vi "超标留样自动校时.vi"   [LabVIEW 2016, in "德润DR803L超标留样.lvlib"]
types:
  T1 = enum16{"open", "read", "write", "write single", "close"}
  T2 = cluster{"采样器状态":enum16{"停止", "运行"}, "当前留样瓶编号":u16, "报警状态":enum16{"无报警", "缺水报警"}, "超标信号":enum16{"无信号", "超标信号"}, "采样器进程":enum16{"停止", "待机", "定位校正", "移除瓶盖", "采样瓶排空", "管路润洗", "管存", "进样", "瓶盖密封", "管路排空", "调整采样位置", "采样结束", "采样瓶润洗", "瓶润洗排空"}, "版本号":string, "同步信号":enum16{"无信号", "同步信号"}, "外控信号":enum16{"无信号", "外控信号"}, "门状态":enum16{"门开", "门关"}, "当前瓶号":u16, "工作状态":enum16{"停止", "采样中"}, "留样模式":enum16{"无", "定时留样", "时间等比例", "超标留样", "同步留样", "外控留样"}, "立即留样":enum16{"无", "远程留样"}, "采样方式":enum16{"单采", "双重"}, "仪器时间":timestamp, "单次采样量":u16, "时间等比采样采样间隔":u16, "排空命令":u16, "远程复位":u16, "门禁密码":u16}
  T3 = typedef "LVDateTimeRec.ctl" = cluster{"秒数的小数部分":dbl, "秒":i32, "分":i32, "时":i32, "日":i32, "月":i32, "年":i32, "天数（周）":i32, "天数（年）":i32, "DST":i32}
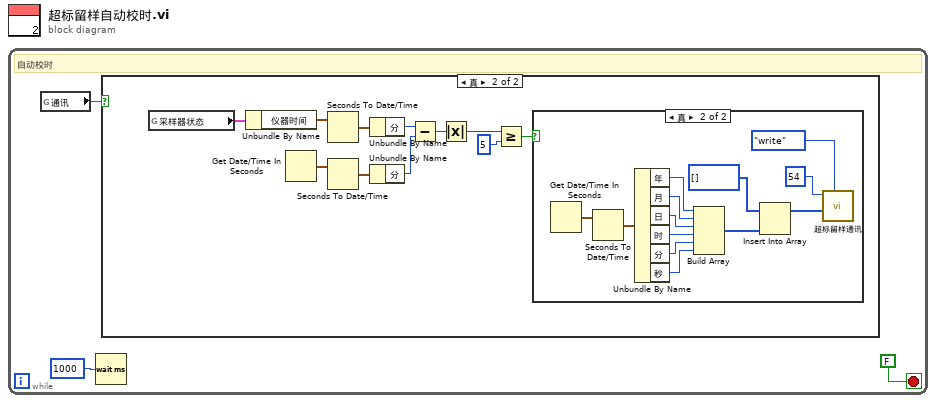
[diagram p0: block diagram]
diagram:
  n1 = while {
    stop <- FALSE stop-if-true
    # "自动校时"
    n2 = global read "超标留样全局.vi" "通讯"() -> (w1:bool)
    n3 = Wait (ms)(milliseconds to wait=u32 1000 ("等待时间（毫秒）")) -> ()  [unwired: 1 out]
    n4 = case shown="真" w1 {
      frame False {
      }
      frame True {
        n5 = global read "超标留样全局.vi" "采样器状态"() -> (w14:T2)
        n6 = Unbundle By Name(w14) -> ("仪器时间"=w13:timestamp)
        n7 = Get Date/Time In Seconds() -> (seconds since 1Jan1904=w11:timestamp)
        n8 = Seconds To Date/Time(time stamp (now)=w13) -> (date time rec=w12:T3)  [unwired: 1 in]
        n9 = Seconds To Date/Time(time stamp (now)=w11) -> (date time rec=w10:T3)  [unwired: 1 in]
        n10 = Unbundle By Name(w12) -> ("分"=w9:i32)
        n11 = Unbundle By Name(w10) -> ("分"=w8:i32)
        n12 = Subtract(x=w9, y=w8) -> (x-y=w6:i32)
        n13 = Absolute Value(x=w6) -> (abs(x)=w5:i32)
        n14 = Greater Or Equal?(x=w5, y=5) -> (x >= y?=w4:bool)
        n15 = case shown="真" w4 {
          frame False {
          }
          frame True {
            n16 = Get Date/Time In Seconds() -> (seconds since 1Jan1904=w15:timestamp)
            n17 = Seconds To Date/Time(time stamp (now)=w15) -> (date time rec=w16:T3)  [unwired: 1 in]
            n18 = Unbundle By Name(w16) -> ("年"=w19:i32, "月"=w20:i32, "日"=w21:i32, "时"=w22:i32, "分"=w23:i32, "秒"=w24:i32)
            n19 = Build Array(w19, w20, w21, w22, w23, w24) -> (w25:i32[])
            n20 = Insert Into Array(array=u16[] [] ("values"), new element=w25) -> (w18:u16[])  [unwired: 1 in]
            n21 = call "超标留样通讯.vi"("STEP"=T1."write", "values"=w18, "starting address"=54 ("索引")) -> ()  [unwired: 6 in, 3 out]
          }
        }
      }
    }
  }
